vi "_PC_RTLoop_Set_Idle.vi"(7 "Function":T1(ring)=enum."writeState", 8 "error in (no error)":errorcluster, 11 "exe_state":bool) -> (0 "error out":errorcluster, 2 "rt_state":bool)   [LabVIEW 2018]
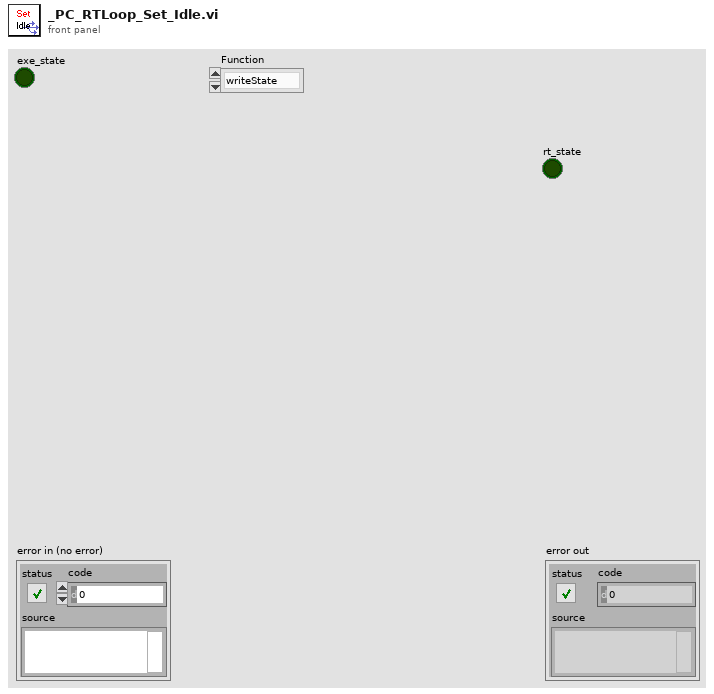
[diagram p1: front panel]
types:
  T1 = enum16{"init", "writeState", "readState", "close"}
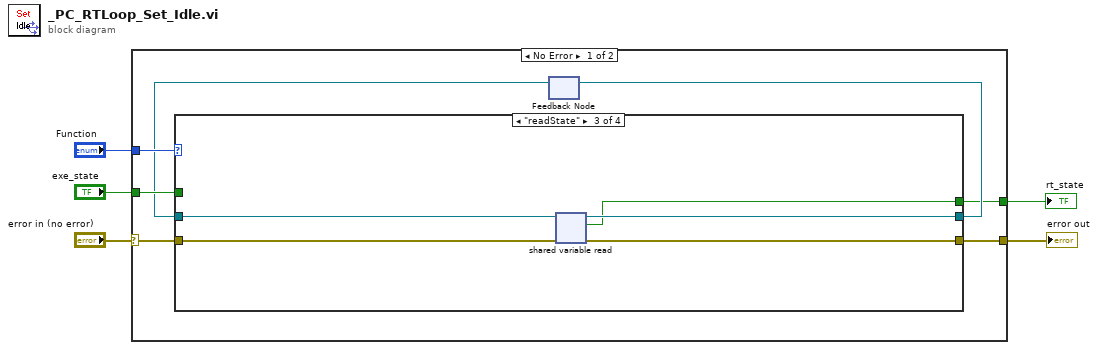
[diagram p0: block diagram]
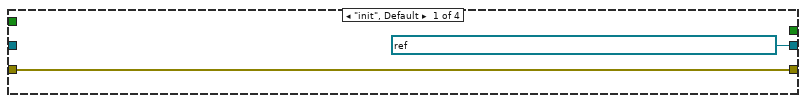
[diagram p2: hidden frame]
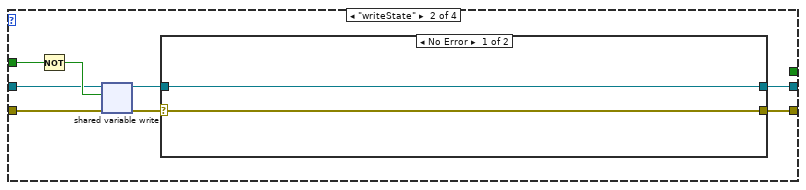
[diagram p3: hidden frame]
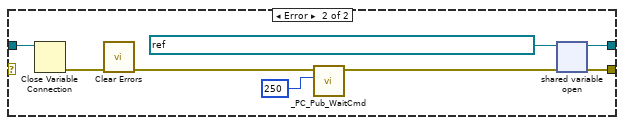
[diagram p4: hidden frame]
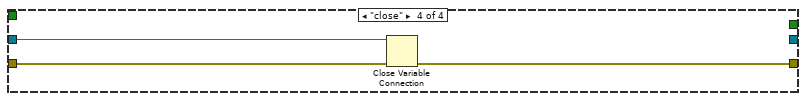
[diagram p5: hidden frame]
diagram:
  n1 = case shown="No Error" "error in (no error)" {
    selector: "error in (no error)" -> [w6 w41]
    tunnel: [w12 w41] -> w5
    tunnel: "Function" -> [w10 _]
    tunnel: "exe_state" -> [w9 _]
    tunnel: [w7 _] -> w2
    frame No Error {
      n2 = feedback #1() -> (w8:refnum<k21>)  [unwired: 1 in]
      n3 = case shown="\"readState\"" w10 {
        tunnel: w6 -> [w13 w21 w35 w40]
        tunnel: [w13 w19 w36 w39] -> w12
        tunnel: [refnum<k21> "ni.var.psp://NI-sbRIO/_RT_CtrlLoop_Safty_Variables/system_idle" ("shared variable refnum in") w17 w37 _] -> w11
        tunnel: w9 -> [_ w16 _ _]
        tunnel: w8 -> [_ w15 w34 w38]
        tunnel: [_ _ w33 _] -> w7
        frame "init", Default {
        }
        frame "writeState" {
          n4 = Not(x=w16) -> (.not. x?=w22:bool)
          n5 = shared-variable-write(w15, w21, w22) -> (w20:refnum<k21>, w18:errorcluster)
          n6 = case shown="No Error" w18 {
            selector: w18 -> [w23 _]
            tunnel: w20 -> [w24 w29]
            tunnel: [w23 w27] -> w19
            tunnel: [w24 w28] -> w17
            frame No Error {
            }
            frame Error {
              n7 = Close Variable Connection(11:w29) -> (0:w32:errorcluster)  [unwired: 1 in]
              n8 = call <vilib>:"Clear Errors.vi"("error in (no error)"=w32) -> ("error out"=w31:errorcluster)  [unwired: 5 in, 1 out]
              n9 = call "_PC_Pub_WaitCmd.vi"("milliseconds to wait"=u32 250, "error in (no error)"=w31) -> ("error out"=w25:errorcluster)  [unwired: 9 in]
              n10 = shared-variable-open(refnum<k21> "ni.var.psp://NI-sbRIO/_RT_CtrlLoop_Safty_Variables/system_idle" ("shared variable refnum in"), w25) -> (w28:refnum<k21>, w27:errorcluster)
            }
          }
        }
        frame "readState" {
          n11 = shared-variable-read(w34, w35) -> (w37:refnum<k21>, w36:errorcluster, w33:bool)  [unwired: 1 out]
        }
        frame "close" {
          n12 = Close Variable Connection(8:w40, 11:w38) -> (0:w39:errorcluster)
        }
      }
      n13 = feedback-in #1(w11) -> ()
    }
    frame Error {
    }
  }
  "error out" <- w5
  "rt_state" <- w2
